vi "THzTime_SPEED_control_for Varying Gap_170222.vi"(1 "ESP300 Axis":i8=1, 2 "ESP300 Address":string="1", 4 "Lockin Address":string="12") -> ()   [LabVIEW 2010]
panel:
  in  "?":bool
  out "Current Round":i32=160
  out "Current Gap (um)":u32=100
  in  "Initial Gap (um)":u32=100
  out "error out":errorcluster
  in  "Number of Gap":u32=8
  in  "Number of Avg":u32=20
  in  "Gap Increase (um)":u32=25
  in  "Step Increase (um)":u32=1
  in  "error in (no error)":errorcluster
  in  "MCS System Locator":string="usb:id:1441320285"
  out "Y position":dbl=-5.0 format="%#.3p"
  out "X position":dbl=-5.0 format="%#.3p"
  out "Power meter":dbl format="%#.3p"
  in  "Save File Name":string="vg_"
  in  "Launch server?":bool
  in  "Authorize?":bool=TRUE
  in  "CONEX-PSD9 Instrument Key 2":string="CONEX-PSD (A6ULD73M)"
  in  "Interdelay (ms)":dbl=20.0
  in  "pre delay(ms)":dbl=300.0
  out "Lock-in Y-Channel":dbl=4.3656e-11 format="%#.3p"
  out "Lock-in X-Channel":dbl=7.4579e-11 format="%#.3p"
  out "THz Time-domain Signal Wave":cluster{"x-axis":sgl[], "y-axis":dbl[]}(graph)
  in  "Autosave Directory for Long-term Average Scan":path=path "D:/taianh/Measurement Data/170204 Variable Gap"
  in  "OK Button":bool
  out "Data Type":string="outp ? 1"
  in  "Enum":enum16{"X", "Y", "Abs"}(ring)
  in  "Draw":bool
  in  "Exit Program":bool
  in  "Short term \nAverage#":i8=1
  in  "Step":sgl=0.005 min=0 max=10000 format="%.3f"
  in  "End Position":sgl=-10.5 min=-75 max=75 format="%#.3f"
  in  "Start Position":sgl=-8.0 min=-75 max=75 format="%#.3f"
  # "Data"
  # "Auto-offset"
  # "Start Position (mm)"
  # "End Position (mm)"
  # "Step (mm)"
  # "Point Avg"
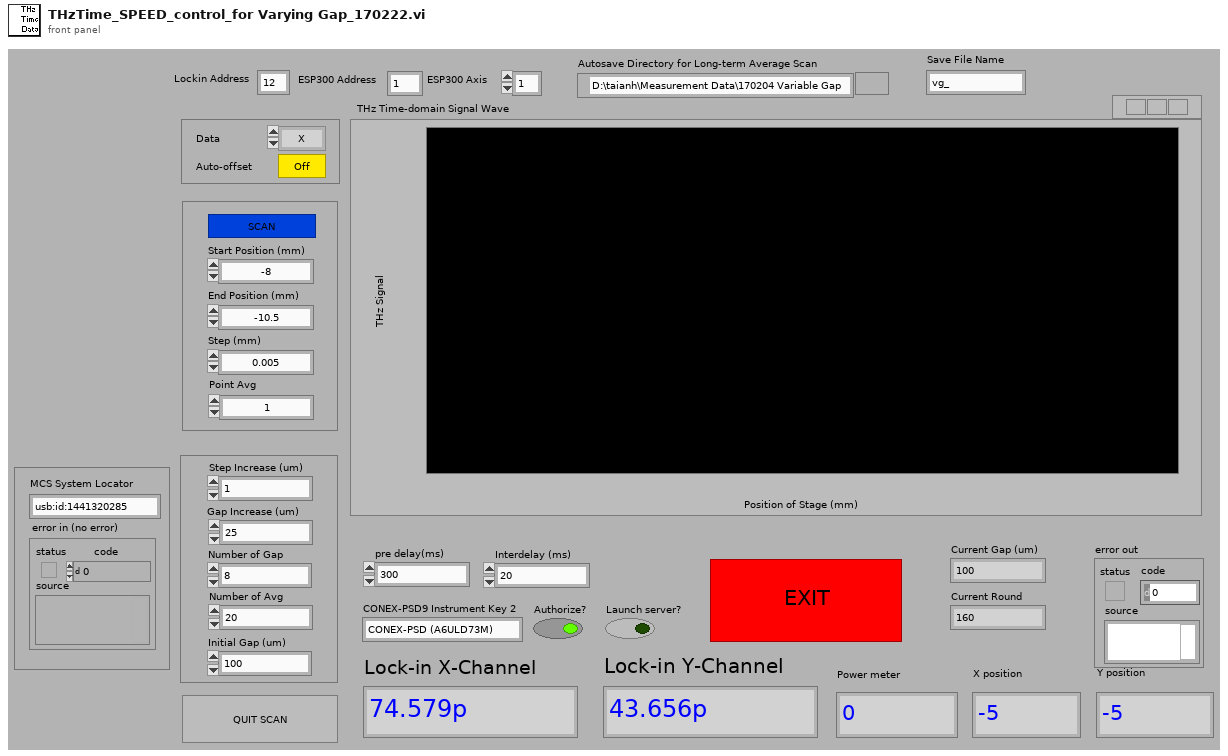
[diagram p1: front panel]
types:
  T1 = cluster{"ConexPSD Reference":refnum<k24>, "error out":errorcluster, "Component ID":i32}
  T2 = cluster{"System Index Out":u32, "error out":errorcluster}
  T3 = cluster{"Step Number":i32, "Step":sgl, "Start Position":sgl, "Time-out":i32, "Lockin Address":string, "Short term \nAverage#":i8, i32, "ESP300 Axis":i8, "Value":string, "pre delay(ms)":dbl, "Interdelay (ms)":dbl, "Autosave Directory for Long-term Average Scan":path, cluster{"ConexPSD Reference":refnum<k24>, "error out":errorcluster, "Component ID":i32}}
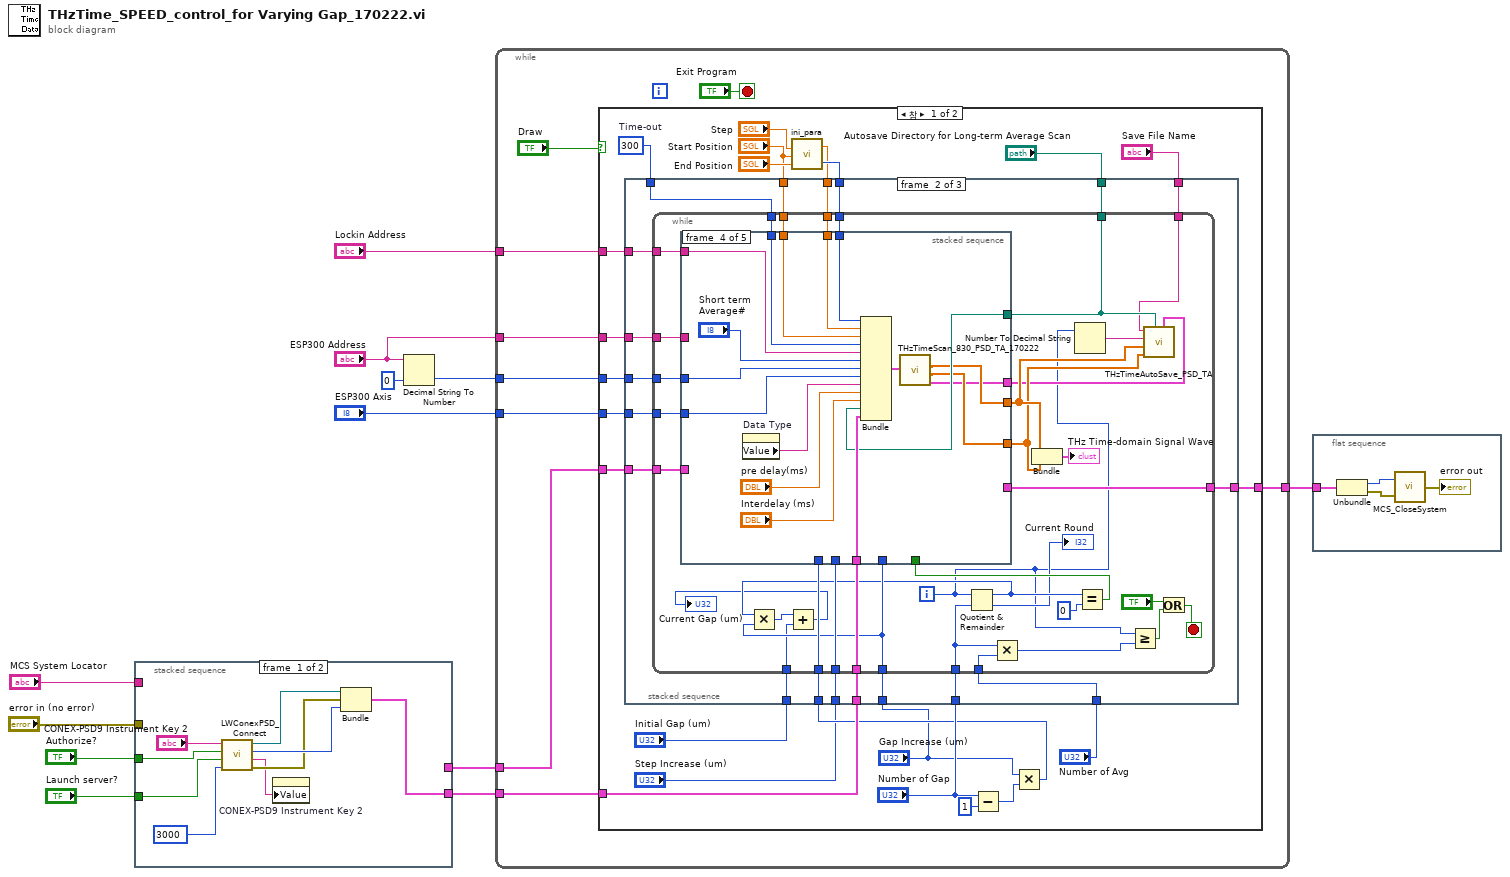
[diagram p0: block diagram]
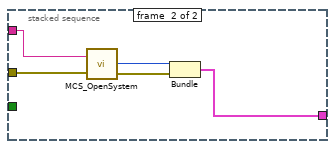
[diagram p2: hidden frame]
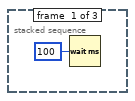
[diagram p3: hidden frame]
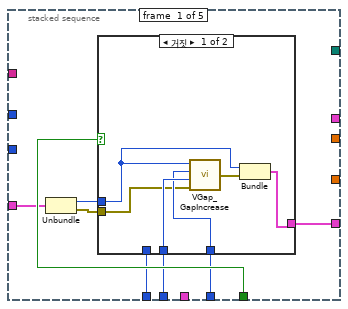
[diagram p4: hidden frame]
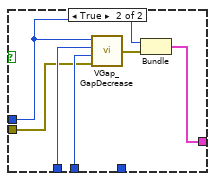
[diagram p5: hidden frame]
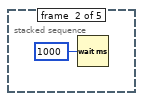
[diagram p6: hidden frame]
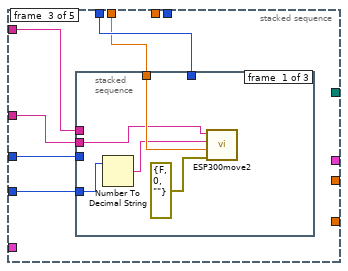
[diagram p7: hidden frame]
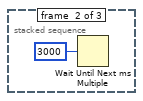
[diagram p8: hidden frame]
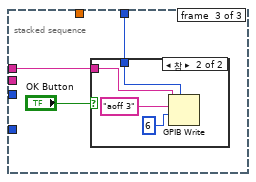
[diagram p9: hidden frame]
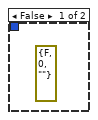
[diagram p10: hidden frame]
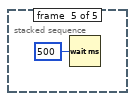
[diagram p11: hidden frame]
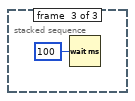
[diagram p12: hidden frame]
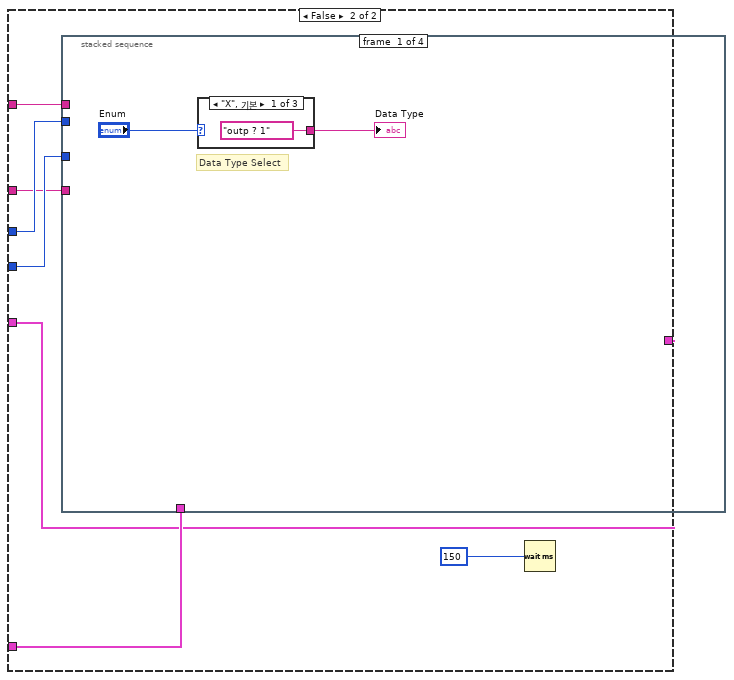
[diagram p13: hidden frame]
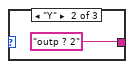
[diagram p14: hidden frame]
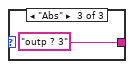
[diagram p15: hidden frame]
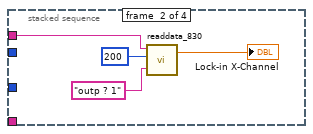
[diagram p16: hidden frame]
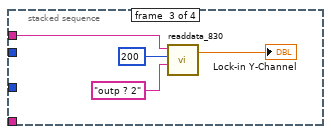
[diagram p17: hidden frame]
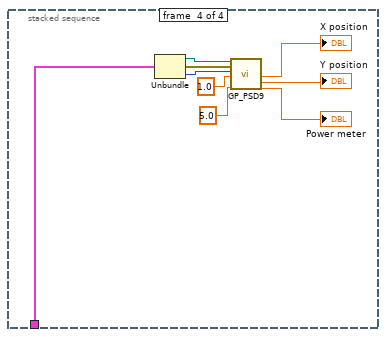
[diagram p18: hidden frame]
diagram:
  n1 = stacked-sequence {
    tunnel: "Authorize?" -> [w15 _]
    tunnel: [w14 _] -> w5
    tunnel: "Launch server?" -> [w13 _]
    tunnel: "MCS System Locator" -> [_ w26]
    tunnel: "error in (no error)" -> [_ w25]
    tunnel: [_ w22] -> w2
    frame #0 {
      n2 = call "LWConexPSD_Connect.vi"("DiscoverTimeout (10000 msec)"=3000, "Launch server? (True)"=w13, "Authorize? (True)"=w15, "Instrument Key"="CONEX-PSD9 Instrument Key 2") -> ("error out"=w19:errorcluster, "Instrument Key out"=w17:string, "Component ID"=w20:i32, "ConexPSD Reference"=w18:refnum<k24>)
      n3 = property on="CONEX-PSD9 Instrument Key 2" class="Str"("Value"=w17) -> ()  [unwired: 2 in, 2 out]
      n4 = Bundle("ConexPSD Reference"=w18, "error out"=w19, "Component ID"=w20) -> (w14:T1)  [unwired: 1 in]
    }
    frame #1 {
      n5 = call "MCS_OpenSystem.vi"("error in (no error)"=w25, "MCS System Locator"=w26) -> ("error out"=w23:errorcluster, "System Index Out"=w24:u32)
      n6 = Bundle("System Index Out"=w24, "error out"=w23) -> (w22:T2)  [unwired: 1 in]
    }
  }
  n7 = Decimal String To Number(string="ESP300 Address", default (0L)=0 ("default (0 I32)")) -> (number=w10:i32)  [unwired: 1 in, 1 out]
  n8 = while {
    tunnel: "ESP300 Axis" -> [w33]
    tunnel: "Lockin Address" -> [w32]
    tunnel: w10 -> [w31]
    tunnel: "ESP300 Address" -> [w30]
    tunnel: w5 -> [w29]
    tunnel: w2 -> [w28]
    tunnel: [w27] -> w1
    stop <- "Exit Program" stop-if-true
    n9 = case shown="참" "Draw" {
      tunnel: w32 -> [w58 w177]
      tunnel: w33 -> [w57 w179]
      tunnel: w31 -> [w56 w178]
      tunnel: w30 -> [w48 w175]
      tunnel: w29 -> [w47 w174]
      tunnel: w28 -> [w46 w173]
      tunnel: [w38 w173] -> w27
      frame True {
        w55 = 300  # Time-out
        n10 = call "ini_para.vi"("End Position"="End Position", "Start Position"="Start Position", "Step"="Step") -> ("Step Number"=w52:i32, "Step"=w51:sgl)
        n11 = Subtract(x="Number of Gap", y=u32 1) -> (x-y=w43:u32)
        n12 = Multiply(x="Gap Increase (um)", y=w43) -> (x*y=w42:u32)
        n13 = stacked-sequence {
          tunnel: w58 -> [_ w78 _]
          tunnel: w55 -> [_ w77 _]
          tunnel: w57 -> [_ w76 _]
          tunnel: w56 -> [_ w75 _]
          tunnel: w52 -> [_ w73 _]
          tunnel: w51 -> [_ w71 _]
          tunnel: "Start Position" -> [_ w74 _]
          tunnel: "Autosave Directory for Long-term Average Scan" -> [_ w72 _]
          tunnel: w48 -> [_ w70 _]
          tunnel: w47 -> [_ w69 _]
          tunnel: "Save File Name" -> [_ w68 _]
          tunnel: "Number of Gap" -> [_ w67 _]
          tunnel: w46 -> [_ w66 _]
          tunnel: w42 -> [_ w65 _]
          tunnel: "Step Increase (um)" -> [_ w64 _]
          tunnel: "Gap Increase (um)" -> [_ w63 _]
          tunnel: "Number of Avg" -> [_ w60 _]
          tunnel: [_ w62 _] -> w38
          tunnel: "Initial Gap (um)" -> [_ w61 _]
          frame #0 {
            n14 = Wait (ms)(milliseconds to wait=u32 100) -> ()  [unwired: 1 out]
          }
          frame #1 {
            n15 = while {
              tunnel: w77 -> [w112]
              tunnel: w78 -> [w113]
              tunnel: w76 -> [w111]
              tunnel: w75 -> [w110]
              tunnel: w74 -> [w109]
              tunnel: w71 -> [w108]
              tunnel: w73 -> [w107]
              tunnel: w72 -> [w100]
              tunnel: w70 -> [w105]
              tunnel: w69 -> [w104]
              tunnel: w68 -> [w99]
              tunnel: w67 -> [w83]
              tunnel: w66 -> [w95]
              tunnel: w65 -> [w92]
              tunnel: w64 -> [w94]
              tunnel: w63 -> [w91]
              tunnel: [w93] -> w62
              tunnel: w61 -> [w89]
              tunnel: w60 -> [w82]
              i -> [w79]
              stop <- w84 stop-if-true
              n16 = Quotient & Remainder(x=w79, y=w83) -> (x-y*floor(x/y)=w90:u32, floor(x/y)=→"Current Round":u32)
              n17 = Multiply(x=w90, y=w91) -> (x*y=w88:u32)
              n18 = Add(x=w88, y=w89) -> (x+y=→"Current Gap (um)":u32)
              n19 = Multiply(x=w83, y=w82) -> (x*y=w81:u32)
              n20 = Number To Decimal String(number=w79) -> (decimal integer string=w103:string)  [unwired: 1 in]
              n21 = Equal?(x=w90, y=u32 0) -> (x = y?=w96:bool)
              n22 = stacked-sequence {
                tunnel: w113 -> [_ _ w140 w166 _]
                tunnel: w112 -> [_ _ w139 w167 _]
                tunnel: w111 -> [_ _ w138 w163 _]
                tunnel: w110 -> [_ _ w137 w164 _]
                tunnel: w109 -> [_ _ w136 w168 _]
                tunnel: w108 -> [_ _ _ w169 _]
                tunnel: w107 -> [_ _ _ w170 _]
                tunnel: [_ _ _ w156 _] -> w102
                tunnel: [_ _ _ w155 _] -> w101
                tunnel: w105 -> [_ _ w135 _ _]
                tunnel: w100 -> [_ _ _ w158 _]
                tunnel: w104 -> [_ _ _ w159 _]
                tunnel: [_ _ _ w154 _] -> w98
                tunnel: w96 -> [w121 _ _ _ _]
                tunnel: w95 -> [w117 _ _ _ _]
                tunnel: w92 -> [w120 _ _ _ _]
                tunnel: w94 -> [w119 _ _ _ _]
                tunnel: w91 -> [w118 _ _ _ _]
                tunnel: [w114 _ _ _ _] -> w93
                frame #0 {
                  n23 = Unbundle(w117) -> ("System Index Out"=w115:u32, "error out"=w116:errorcluster)
                  n24 = case shown="거짓" w121 {
                    tunnel: w120 -> [_ w133]
                    tunnel: w119 -> [w127 w132]
                    tunnel: w118 -> [w126 _]
                    tunnel: w115 -> [w123 w129]
                    tunnel: w116 -> [w125 w131]
                    tunnel: [w122 w128] -> w114
                    frame False {
                      n25 = call "VGap_GapIncrease.vi"("error in (no error)"=w125, "Step Increase (um)"=w127, "Gap Increase (um)"=w126, "System Index In"=w123) -> ("error out"=w124:errorcluster)
                      n26 = Bundle("System Index Out"=w123, "error out"=w124) -> (w122:T2)  [unwired: 1 in]
                    }
                    frame True {
                      n27 = call "VGap_GapDecrease.vi"("error in (no error)"=w131, "Step Decrease (um)"=w132, "Gap Decrease (um)"=w133, "System Index In"=w129) -> ("error out"=w130:errorcluster)
                      n28 = Bundle("System Index Out"=w129, "error out"=w130) -> (w128:T2)  [unwired: 1 in]
                    }
                  }
                }
                frame #1 {
                  n29 = Wait (ms)(milliseconds to wait=u32 1000 ("대기 시간(ms)")) -> ()  [unwired: 1 out]
                }
                frame #2 {
                  n30 = stacked-sequence {
                    tunnel: w140 -> [_ _ w148]
                    tunnel: w139 -> [_ _ w147]
                    tunnel: w138 -> [w142 _ _]
                    tunnel: w137 -> [_ _ _]
                    tunnel: w136 -> [w145 _ _]
                    tunnel: w135 -> [w143 _ _]
                    frame #0 {
                      n31 = Number To Decimal String(number=w142) -> (decimal integer string=w141:string)  [unwired: 1 in]
                      n32 = call "ESP300move2.vi"("ESP300 Address"=w143, "ESP300 Channel"=w141, "Target"=w145, "error in (no error) 2"=errorcluster {"status"=FALSE, "code"=0, "source"=""}) -> ()  [unwired: 6 in, 1 out]
                    }
                    frame #1 {
                      n33 = Wait Until Next ms Multiple(millisecond multiple=3000) -> ()  [unwired: 1 out]
                    }
                    frame #2 {
                      n34 = case shown="참" "OK Button" {
                        tunnel: w148 -> [_ w153]
                        tunnel: w147 -> [_ w151]
                        frame False {
                          (unwired) errorcluster {"status"=FALSE, "code"=0, "source"=""} ("error in")
                        }
                        frame True {
                          n35 = GPIB Write(0:w153, 1:"aoff 3" ("data"), 2:i16 6 ("mode (0)"), 4:w151) -> ()  [unwired: 1 in, 2 out]
                        }
                      }
                    }
                  }
                }
                frame #3 {
                  n36 = property on="Data Type" class="Str"() -> ("Value"=w162:string)  [unwired: 2 in, 2 out]
                  n37 = Bundle("Step Number"=w170, "Step"=w169, "Start Position"=w168, "Time-out"=w167, "Lockin Address"=w166, "Short term \nAverage#"="Short term \nAverage#", w164, "ESP300 Axis"=w163, "Value"=w162, "pre delay(ms)"="pre delay(ms)", "Interdelay (ms)"="Interdelay (ms)", "Autosave Directory for Long-term Average Scan"=w158, w159) -> (w157:T3)  [unwired: 1 in]
                  n38 = call "THzTimeScan_830_PSD_TA_170222.vi"("input"=w157) -> ("x-axis"=w156:sgl[], "y-axis"=w155:dbl[], "ext. out"=w154:cluster{dbl[], dbl[], dbl[], dbl[], string[]})  [unwired: 1 out]
                }
                frame #4 {
                  n39 = Wait (ms)(milliseconds to wait=u32 500) -> ()  [unwired: 1 out]
                }
              }
              n40 = Bundle("x-axis"=w102, "y-axis"=w101) -> (→"THz Time-domain Signal Wave":cluster{"x-axis":sgl[], "y-axis":dbl[]})  [unwired: 1 in]
              n41 = Greater Or Equal?(x=w79, y=w81) -> (x >= y?=w85:bool)
              n42 = call "THzTimeAutoSave_PSD_TA.vi"("ext. out"=w98, "Autosave Directory for Long-term Average Scan"=w100, "y-axis"=w101, "x-axis"=w102, "String"=w103, "SaveFile name"=w99) -> ()  [unwired: 4 in]
              n43 = Or(x="?", y=w85) -> (x .or. y?=w84:bool)
            }
          }
          frame #2 {
            n44 = Wait (ms)(milliseconds to wait=u32 100) -> ()  [unwired: 1 out]
          }
        }
      }
      frame False {
        n45 = stacked-sequence {
          tunnel: w179 -> [_ _ _ _]
          tunnel: w178 -> [_ _ _ _]
          tunnel: w177 -> [_ w188 w192 _]
          tunnel: w175 -> [_ _ _ _]
          tunnel: w174 -> [_ _ _ w193]
          frame #0 {
            # "Data Type Select"
            n46 = case shown="\"X\", 기본" "Enum" {
              tunnel: ["outp ? 1" "outp ? 2" "outp ? 3"] -> w181
              frame "X", Default {
              }
              frame "Y" {
              }
              frame "Abs" {
              }
            }
            "Data Type" <- w181
          }
          frame #1 {
            n47 = call "readdata_830.vi"("Command"="outp ? 1", "timeout"=200, "Lockin Address"=w188) -> ("Data"=→"Lock-in X-Channel":dbl)  [unwired: 1 in, 1 out]
          }
          frame #2 {
            n48 = call "readdata_830.vi"("Command"="outp ? 2", "timeout"=200, "Lockin Address"=w192) -> ("Data"=→"Lock-in Y-Channel":dbl)  [unwired: 1 in, 1 out]
          }
          frame #3 {
            n49 = Unbundle(w193) -> ("ConexPSD Reference"=w201:refnum<k24>, "error out"=w200:errorcluster, "Component ID"=w199:i32)
            n50 = call "GP_PSD9.vi"("ConexPSD Reference"=w201, "error out"=w200, "Component ID"=w199, "Adress"=1.0 ("shot average"), "shot average"=5.0) -> ("PositionX"=→"X position":dbl, "PositionY"=→"Y position":dbl, "LaserPower"=→"Power meter":dbl)  [unwired: 8 in, 4 out]
          }
        }
        n51 = Wait (ms)(milliseconds to wait=u32 150) -> ()  [unwired: 1 out]
      }
    }
  }
  n52 = flat-sequence {
    tunnel: w1 -> [w205]
    frame #0 {
      n53 = Unbundle(w205) -> ("System Index Out"=w204:u32, "error out"=w203:errorcluster)
      n54 = call "MCS_CloseSystem.vi"("error in (no error)"=w203, "System Index In"=w204) -> ("error out"=→"error out":errorcluster)
    }
  }
